vi "Get BURST.vi"(8 "error in (no error)":errorcluster, 10 "chan (0)":i32, 11 "VISA resource name":refnum<visa-resource-name>) -> (0 "error out":errorcluster, 1 "subarray":dbl[](array[numeric]), 3 "VISA resource name out":refnum<visa-resource-name>, 4 "return count":u32)   [LabVIEW 2025, in "Detector SCPI.lvlib"]
doc: "Gets burst of data from ADC\nData size is set by OS level"
uses:
  Detector SCPI.lvlib
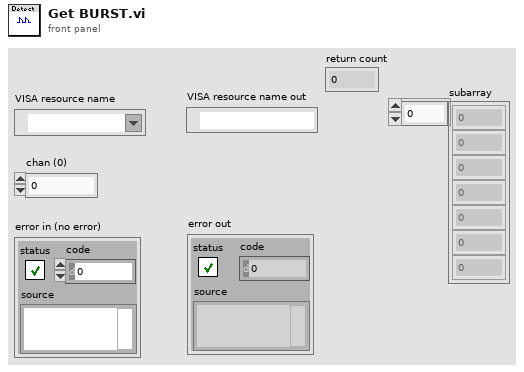
[diagram p1: front panel]
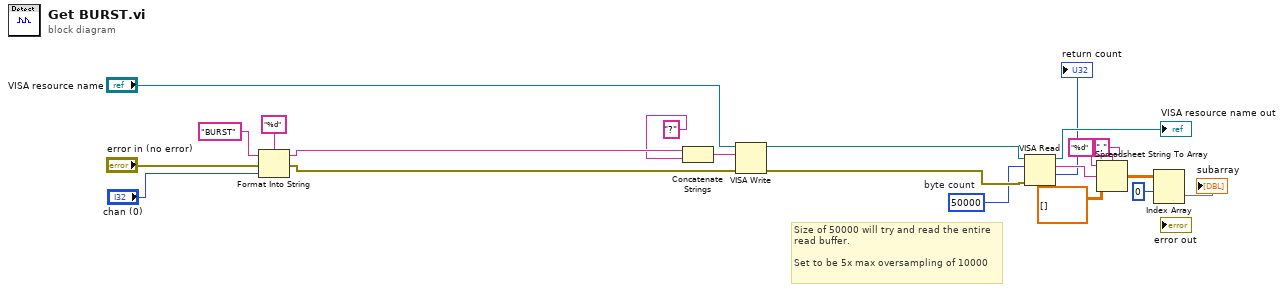
[diagram p0: block diagram]
diagram:
  w10 = u32 50000  # byte count
  # "Size of 50000 will try and read the entire\nread buffer.\n\nSet to be 5x max oversampling of 10000"
  n1 = Format Into String(format string="%d", initial string="BURST" ("command"), error in="error in (no error)", "chan (0)") -> (resulting string=w13:string, error out=w19:errorcluster)
  n2 = Concatenate Strings(w13, "?" ("command")) -> (w14:string)
  n3 = VISA Write(VISA resource name="VISA resource name", write buffer=w14, error in (no error)=w19) -> (VISA resource name out=w9:refnum<visa-resource-name>, error out=w15:errorcluster)  [unwired: 1 out]
  n4 = VISA Read(VISA resource name=w9, byte count=w10, error in (no error)=w15) -> (VISA resource name out=→"VISA resource name out":refnum<visa-resource-name>, read buffer=w8:string, return count=→"return count":u32)  [unwired: 1 out]
  n5 = Spreadsheet String To Array(delimiter (Tab)=",", format string="%d", spreadsheet string=w8, array type (2D Dbl)=dbl[][] []) -> (array=w4:dbl[][])
  n6 = Index Array(array=w4, index (row)=0) -> (element=→"subarray":dbl[])  [unwired: 1 in]
